vi "Elapsed_time.vi"() -> ()   [LabVIEW 2020]
doc: "Oblicza ca³kowity czas gdy nawet pojazd nie jest na poprawnej pozycji."
panel:
  in  "Numeric":dbl
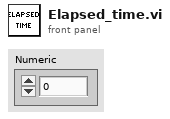
[diagram p1: front panel]
diagram:
